vi "Fit VI window to Content.vi"(4 "error in (no error)":errorcluster, 6 "border spacing (2 px)":i32=2, 7 "VI Ref (calling VI)":refnum<vi>) -> (0 "error out":errorcluster, 3 "dup VI Ref":refnum<vi>)   [LabVIEW 2020]
doc: "This utility will fit (resize and center) a VI (defined by the \"VI Ref\" input) about the all of the Front Panel object. It will add a border defined by border spacing in units of pixels. If no VI Reference is passed in, it will operate on the calling VI."
uses:
  <vilib>/Utility/miscctls.llb/LVPointTypeDef.ctl
panel:
  # "Fit VI window to Content.vi\n\nFits a VI's front panel window to its FP Contents.\n\nPlease visit http://www.OpenG.org to learn about the\nOpen Source LabVIEW software movement.\n\nNOTICE -- YOU MUST LEAVE THIS NOTICE IN PLACE.  PER THE TERMS OF THE LICENSE BELOW, YOU MAY SUBLICENSE THIS SOFTWARE \nIN ANY WAY THAT DOES NOT CONFLICT WITH THIS LICENSE.\n\n### BSD License (http://www.opensource.org/licenses/bsd-license.php) Begin ###\n \nCopyright (c) 2002-2004, Jim Kring <jim@jimkring.com>\nCopyright (c) 2002, Cal-Bay Systems, Inc. <info@calbay.com>\n\nAll rights reserved.\n\nRedistribution and use in source and binary forms, with or without modification, are permitted provided that the following conditions are met:\n\n    * Redistributions of source code must retain the above copyright notice, this list of conditions and the following disclaimer.\n    * Redistributions in binary form must reproduce the above copyright notice, this list of conditions and the following disclaimer in the \n       documentation and/or other materials provided with the distribution.\n    * Neither the name of SciWare, James Kring, Inc., nor the names of its contributors may be used to endorse or promote products derived \n       from this software without specific prior written permission.\n\nTHIS SOFTWARE IS PROVIDED BY THE COPYRIGHT HOLDERS AND CONTRIBUTORS \"AS IS\" AND ANY EXPRESS OR IMPLIED WARRANTIES, \nINCLUDING, BUT NOT LIMITED TO, THE IMPLIED WARRANTIES OF MERCHANTABILITY AND FITNESS FOR A PARTICULAR PURPOSE ARE \nDISCLAIMED. IN NO EVENT SHALL THE COPYRIGHT OWNER OR CONTRIBUTORS BE LIABLE FOR ANY DIRECT, INDIRECT, INCIDENTAL,\n SPECIAL, EXEMPLARY, OR CONSEQUENTIAL DAMAGES (INCLUDING, BUT NOT LIMITED TO, PROCUREMENT OF SUBSTITUTE GOODS OR \nSERVICES; LOSS OF USE, DATA, OR PROFITS; OR BUSINESS INTERRUPTION) HOWEVER CAUSED AND ON ANY THEORY OF LIABILITY, \nWHETHER IN CONTRACT, STRICT LIABILITY, OR TORT (INCLUDING NEGLIGENCE OR OTHERWISE) ARISING IN ANY WAY OUT OF THE USE \nOF THIS SOFTWARE, EVEN IF ADVISED OF THE POSSIBILITY OF SUCH DAMAGE.\n\n### BSD License End ###"
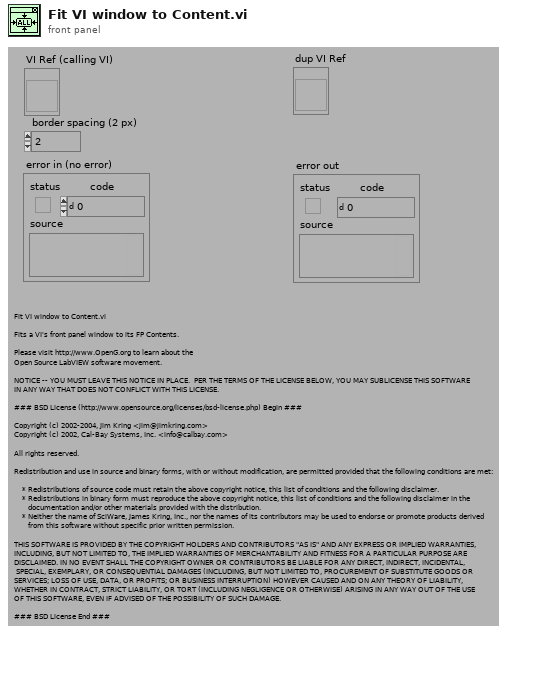
[diagram p1: front panel]
types:
  T1 = typedef "LVPointTypeDef.ctl" = cluster{"Horizontal":i16, "Vertical":i16}
  T2 = typedef "LVRectTypeDef.ctl" = cluster{"Left":i16, "Top":i16, "Right":i16, "Bottom":i16}
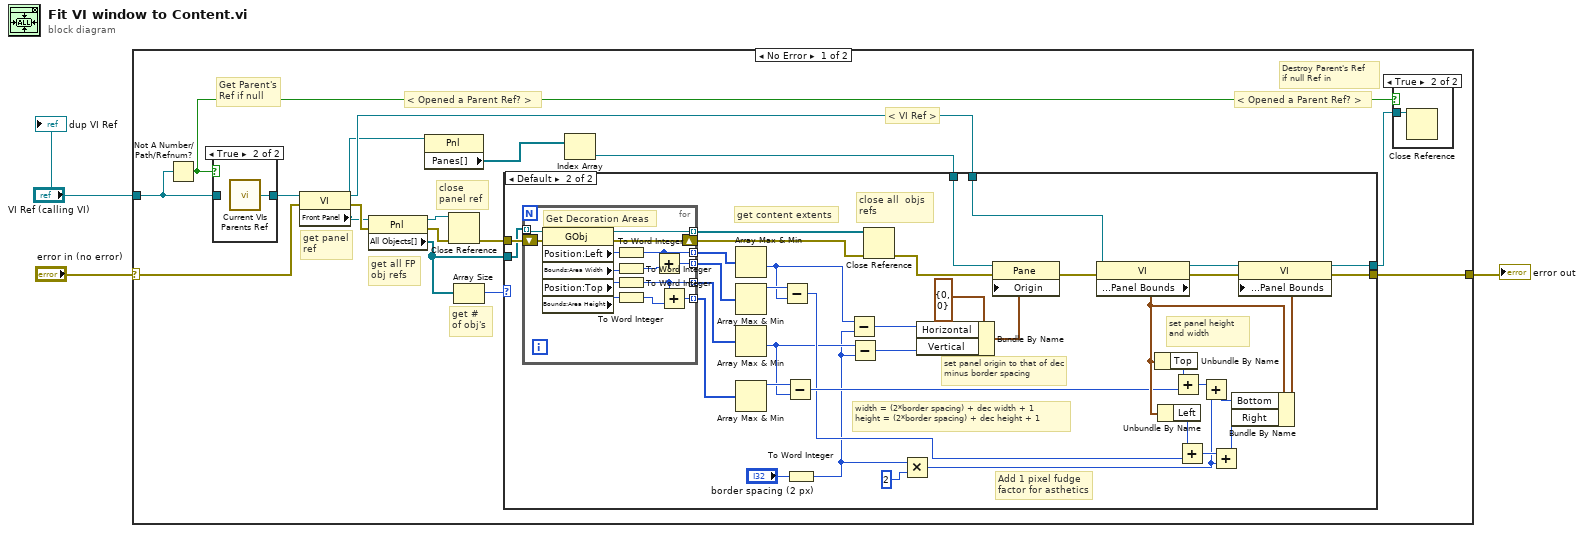
[diagram p0: block diagram]
diagram:
  n1 = case shown="No Error" "error in (no error)" {
    selector: "error in (no error)" -> [w7 w77]
    tunnel: [w14 w77] -> w3
    tunnel: "VI Ref (calling VI)" -> [w8 _]
    frame No Error {
      # "< Opened a Parent Ref? >"
      # "< Opened a Parent Ref? >"
      # "Destroy Parent's Ref\nif null Ref in"
      # "Get Parent's\nRef if null"
      # "get # of obj's"
      # "get panel ref"
      # "get all FP obj refs"
      # "close panel ref"
      # "< VI Ref >"
      n2 = Not A Number/Path/Refnum?(number/path/refnum=w8) -> (NaN/Path/Refnum?=w10:bool)
      n3 = case shown="True" w10 {
        tunnel: [w21 w22] -> w11
        tunnel: w8 -> [w21 _]
        frame False {
        }
        frame True {
          n4 = call "Current VIs Parents Ref.vi"() -> ("Calling VI's reference"=w22:refnum<vi>)  [unwired: 2 in]
        }
      }
      n5 = property on="Property Node" class="VI"(reference=w11, error in=w7) -> (reference out=w19:refnum<vi>, error out=w17:errorcluster, "Front Panel"=w6:refnum<vi>)
      n6 = property on="Property Node" class="Pnl"(reference=w6, error in=w17) -> (reference out=w18:refnum<vi>, error out=w16:errorcluster, "All Objects[]"=w13:refnum<vi>[])
      n7 = property on="Property Node" class="Pnl"(reference=w6) -> ("Panes[]"=w5:refnum<vi>[])  [unwired: 1 in, 2 out]
      n8 = Close Reference(reference=w18, error in (no error)=w16) -> (error out=w15:errorcluster)
      n9 = Array Size(array=w13) -> (size(s)=w12:i32)
      n10 = Index Array(array=w5) -> (element=w4:refnum<vi>)  [unwired: 1 in]
      n11 = case shown="Default" w12 {
        tunnel: w19 -> [w24 w30]
        tunnel: w15 -> [w23 w51]
        tunnel: [w23 w47] -> w14
        tunnel: [w24 w46] -> w9
        tunnel: w13 -> [_ w45]
        tunnel: w4 -> [_ w29]
        frame 0 {
          # "do nothing if no objects"
        }
        frame Default {
          # "width = (2*border spacing) + dec width + 1\nheight = (2*border spacing) + dec height + 1"
          # "set panel height and width"
          # "set panel origin to that of dec minus border spacing"
          # "close all  objs refs"
          # "get content extents"
          # "Add 1 pixel fudge factor for asthetics"
          n12 = for {
            tunnel: w45 -> [w76] mode=indexing
            shift-right: [w74] -> w32
            shift-left: w51 -> [w75]
            tunnel: [w73] -> w33 mode=indexing
            tunnel: [w69] -> w43 mode=indexing
            tunnel: [w71] -> w42 mode=indexing
            tunnel: [w65] -> w41 mode=indexing
            tunnel: [w70] -> w40 mode=indexing
            # "Get Decoration Areas"
            n13 = property class="GObj"(reference=w76, error in=w75) -> (reference out=w73:refnum<vi>, error out=w74:errorcluster, "Position:Left"=w72:i32, "Bounds:Area Width"=w68:u32, "Position:Top"=w66:i32, "Bounds:Area Height"=w64:u32)
            n14 = To Word Integer(number=w72) -> (16bit integer=w69:i16)
            n15 = To Word Integer(number=w68) -> (16bit integer=w67:i16)
            n16 = To Word Integer(number=w66) -> (16bit integer=w65:i16)
            n17 = To Word Integer(number=w64) -> (16bit integer=w63:i16)
            n18 = Add(x=w69, y=w67) -> (x+y=w71:i16)
            n19 = Add(x=w65, y=w63) -> (x+y=w70:i16)
          }
          n20 = Array Max & Min(array=w43) -> (min value=w34:i16)  [unwired: 3 out]
          n21 = Array Max & Min(array=w42) -> (max value=w37:i16)  [unwired: 3 out]
          n22 = Array Max & Min(array=w41) -> (min value=w35:i16)  [unwired: 3 out]
          n23 = Array Max & Min(array=w40) -> (max value=w39:i16)  [unwired: 3 out]
          n24 = Subtract(x=w37, y=w34) -> (x-y=w36:i16)
          n25 = Subtract(x=w39, y=w35) -> (x-y=w38:i16)
          n26 = To Word Integer(number="border spacing (2 px)") -> (16bit integer=w31:i16)
          n27 = Subtract(x=w34, y=w31) -> (x-y=w52:i16)
          n28 = Subtract(x=w35, y=w31) -> (x-y=w53:i16)
          n29 = Close Reference(reference=w33, error in (no error)=w32) -> (error out=w28:errorcluster)
          n30 = Multiply(x=w31, y=i16 2) -> (x*y=w44:i16)
          n31 = Bundle By Name(cluster=T1 {"Horizontal"=0, "Vertical"=0} ("Origin"), "Horizontal"=w52, "Vertical"=w53) -> (w26:T1)
          n32 = property on="Property Node" class="Pane"(reference=w29, error in=w28, "Origin"=w26) -> (error out=w27:errorcluster)  [unwired: 1 out]
          n33 = property on="Property Node" class="VI"(reference=w30, error in=w27) -> (reference out=w62:refnum<vi>, error out=w48:errorcluster, "Front Panel Window:Panel Bounds"=w54:T2)
          n34 = Unbundle By Name(w54) -> ("Top"=w55:i16)
          n35 = Unbundle By Name(w54) -> ("Left"=w56:i16)
          n36 = Add(x=w55, y=w38) -> (x+y=w60:i16)
          n37 = Add(x=w56, y=w36) -> (x+y=w58:i16)
          n38 = Add(x=w60, y=w44) -> (x+y=w61:i16)
          n39 = Add(x=w58, y=w44) -> (x+y=w59:i16)
          n40 = Bundle By Name(cluster=w54, "Bottom"=w61, "Right"=w59) -> (w57:T2)
          n41 = property on="Property Node" class="VI"(reference=w62, error in=w48, "Front Panel Window:Panel Bounds"=w57) -> (reference out=w46:refnum<vi>, error out=w47:errorcluster)
        }
      }
      n42 = case shown="True" w10 {
        tunnel: w9 -> [_ w20]
        frame False {
        }
        frame True {
          n43 = Close Reference(reference=w20) -> ()  [unwired: 1 in, 1 out]
        }
      }
    }
    frame Error {
    }
  }
  "error out" <- w3
  "dup VI Ref" <- "VI Ref (calling VI)"
